vi "Formula node.vi"() -> ()   [LabVIEW 2020]
panel:
  out "Farenheit":dbl
  in  "Celsius":dbl
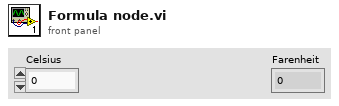
[diagram p1: front panel]
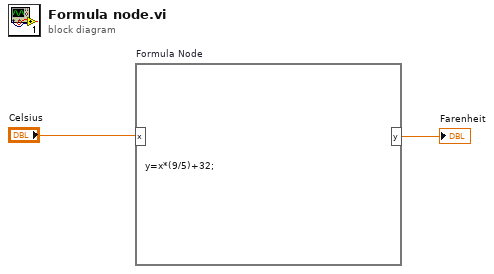
[diagram p0: block diagram]
diagram:
  n1 = formula code="y=x*(9/5)+32;"("x"="Celsius") -> ("y"=→"Farenheit":dbl)
